vi "ReadTubeCorrnFile.vi"(11 "PathToFile":path) -> (2 "F-CompArray":dbl[][](array[numeric]))   [LabVIEW 2016]
panel:
  out "FileContents":string
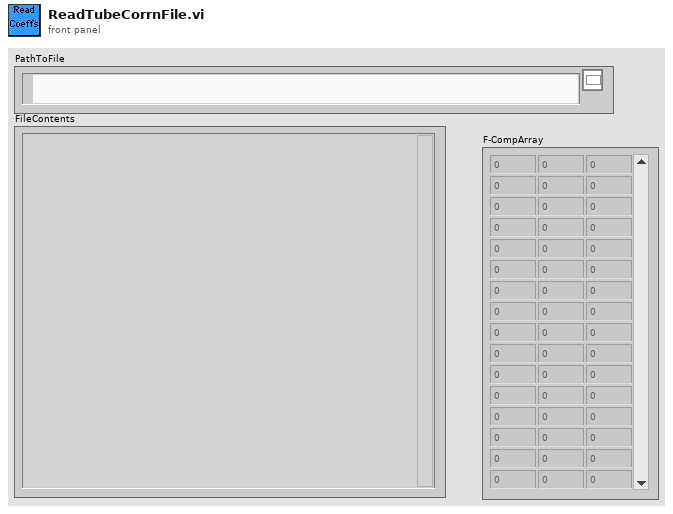
[diagram p1: front panel]
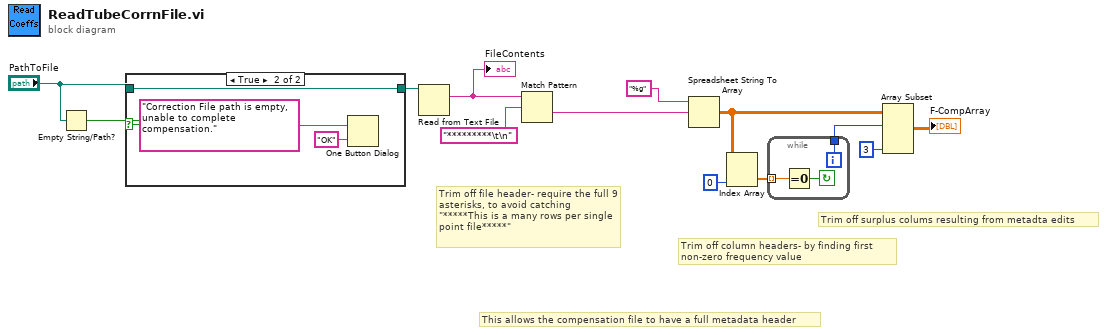
[diagram p0: block diagram]
diagram:
  # "Trim off surplus colums resulting from metadta edits"
  # "This allows the compensation file to have a full metadata header"
  # "This allows the compensation file to have a full metadata header"
  # "Trim off file header- require the full 9 asterisks, to avoid catching \"*****This is a many rows per single point file*****\""
  # "Trim off column headers- by finding first non-zero frequency value"
  n1 = Empty String/Path?(string/path="PathToFile") -> (empty?=w10:bool)
  n2 = case shown="True" w10 {
    tunnel: "PathToFile" -> [w14 w17]
    tunnel: [w14 w17] -> w8
    frame False {
    }
    frame True {
      n3 = One Button Dialog(message="Correction File path is empty, unable to complete compensation.", button name ("OK")="OK") -> ()  [unwired: 1 out]
    }
  }
  n4 = Read from Text File(file (use dialog)=w8) -> (text=w13:string)  [unwired: 3 in, 3 out]
  "FileContents" <- w13
  n5 = Match Pattern(string=w13, regular expression="*********\t\n") -> (after substring=w7:string)  [unwired: 1 in, 3 out]
  n6 = Spreadsheet String To Array(format string="%g", spreadsheet string=w7) -> (array=w4:dbl[][])  [unwired: 2 in]
  n7 = Index Array(array=w4, index (col)=0 ("disabled index (col)")) -> (element=w5:dbl[])  [unwired: 1 in]
  n8 = while {
    tunnel: w5 -> [w20] mode=indexing
    tunnel: [w18] -> w3
    i -> [w18]
    stop <- w19 continue-if-true
    n9 = Equal To 0?(x=w20) -> (x = 0?=w19:bool)
  }
  n10 = Array Subset(array=w4, index (row)=w3, length (col)=3 ("length")) -> (→"F-CompArray":dbl[][])  [unwired: 2 in]
